vi "ControlFoco.vi"() -> ()   [LabVIEW 2018]
panel:
  in  "stop":bool
  out "Foco":bool
  in  "Apagar":bool
  in  "Encender":bool
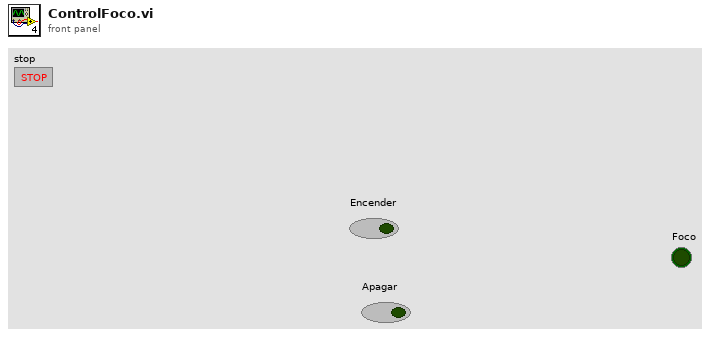
[diagram p1: front panel]
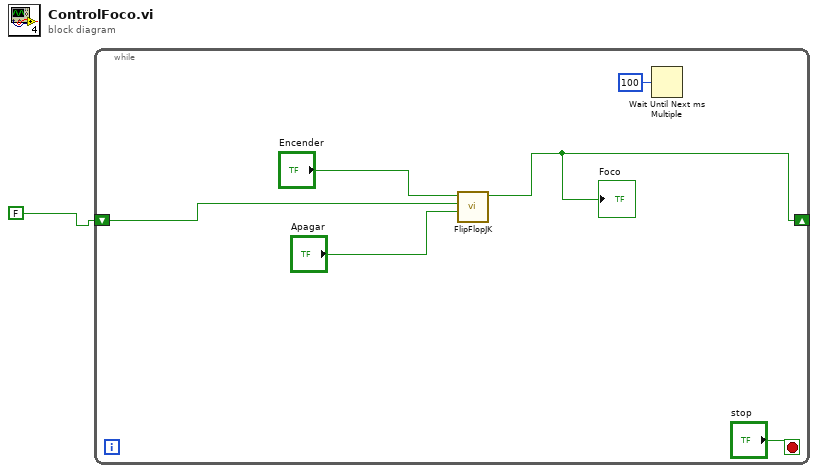
[diagram p0: block diagram]
diagram:
  n1 = while {
    shift-right: [w2] -> _
    shift-left: FALSE -> [w3]
    stop <- "stop" stop-if-true
    n2 = call "FlipFlopJK.vi"("K"="Apagar", "Boolean in"=w3, "J"="Encender") -> ("Boolean out"=w2:bool)  [unwired: 7 in, 1 out]
    "Foco" <- w2
    n3 = Wait Until Next ms Multiple(millisecond multiple=u32 100) -> ()  [unwired: 1 out]
  }
